vi "UDPSend.vi"(4 "error in (no error)":errorcluster, 6 "Data String":string="<data>", 8 "# Repetitions":i32=1, 9 "Remote Port":u16=1234, 10 "Local Port":u16=1233, 11 "Remote Host":string="localhost") -> (0 "error out":errorcluster)   [LabVIEW 2014]
doc: "This VI is designed to be used with the UDP Receiver VI. Run the UDP Receiver.vi first.\n\nThe UDP protocol differs from TCP in that there is no error-checking with the packets of information that are sent, and thus no guarantee whatsoever that an intended recipient will actually receive a given piece of data.\n\nUDP does offer the ability to \"broadcast\" data across a network--simply specify an IP Address of all ones (255.255.255.255) to attempt to broadcast information network-wide. Keep in mind that routers and other network hardware will generally refuse to forward the broadcast beyond certain points, so the extent of the broadcast will in practice be limited."
panel:
  in  "local Host":string="192.168.1.1"
  in  "broadcast":bool
  # "Instructions:\n1. Open the UDP Receiver.vi located in the same library.\n2. Make sure that the Remote Port in this VI and the Port in the UDP Receive.vi are the same.\n3. Press the button if you want to broadcast the data to all the network, instead of sending it to a specific address.\n4. Change the number of times you want to send the data to the receiver in the # of Repetitions control.\n5. Follow the instructions on it's front panel.\nNote: This VI is built to work with the UDP Receiver.vi."
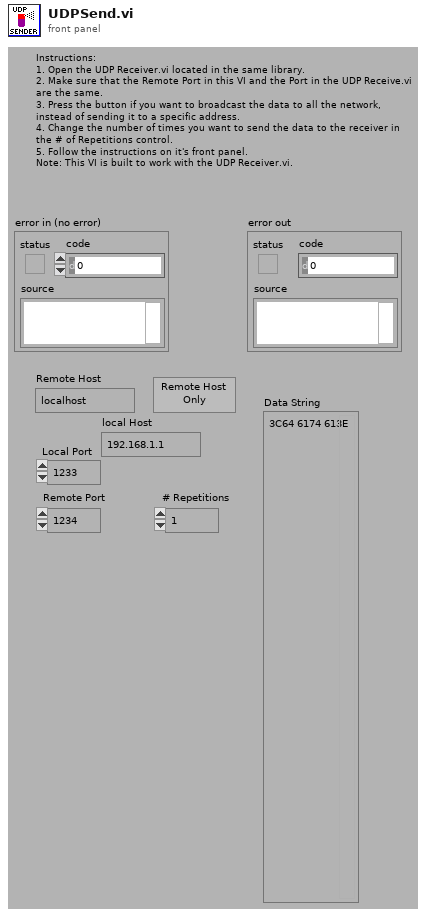
[diagram p1: front panel]
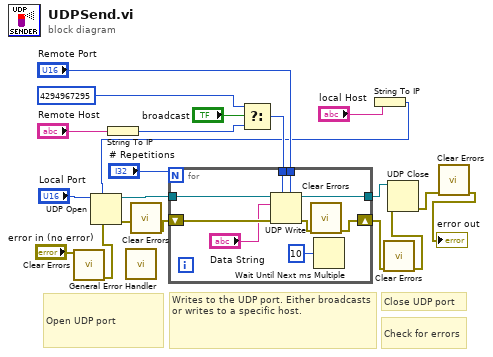
[diagram p0: block diagram]
diagram:
  # "Close UDP port"
  # "Check for errors"
  # "Writes to the UDP port. Either broadcasts or writes to a specific host."
  # "Open UDP port"
  n1 = call <vilib>:"Clear Errors.vi"("error in (no error)"="error in (no error)") -> ("error out"=w7:errorcluster)  [unwired: 1 in, 5 out]
  n2 = String To IP(1:"Remote Host") -> (0:w15:u32)
  n3 = call <vilib>:"General Error Handler.vi"() -> ()  [unwired: 3 in, 13 out]
  n4 = Select(t=u32 4294967295, s="broadcast", f=w15) -> (s? t:f=w14:u32)
  n5 = String To IP(1:"local Host") -> (0:w9:u32)
  n6 = UDP Open(7:w9, 8:w7, 11:"Local Port") -> (port=w20:refnum<k16>, 0:w4:errorcluster)  [unwired: 3 out]
  n7 = call <vilib>:"Clear Errors.vi"("error in (no error)"=w4) -> ("error out"=w3:errorcluster)  [unwired: 1 in, 5 out]
  n8 = for {
    N: "# Repetitions" -> [_]
    tunnel: w20 -> [w27]
    tunnel: w14 -> [w29]
    tunnel: "Remote Port" -> [w28]
    shift-right: [w21] -> w6
    shift-left: w3 -> [w26]
    tunnel: [w25] -> w18
    n9 = UDP Write(address=w29, port or service name=w28, connection ID=w27, data in="Data String", 8:w26) -> (error out=w22:errorcluster, 3:w25:refnum<k16>)  [unwired: 1 out]
    n10 = call <vilib>:"Clear Errors.vi"("error in (no error)"=w22) -> ("error out"=w21:errorcluster)  [unwired: 1 in, 5 out]
    n11 = Wait Until Next ms Multiple(millisecond multiple=u32 10) -> ()  [unwired: 1 out]
  }
  n12 = call <vilib>:"Clear Errors.vi"("error in (no error)"=w6) -> ("error out"=w5:errorcluster)  [unwired: 1 in, 5 out]
  n13 = UDP Close(connection ID=w18, 8:w5) -> (error out=w2:errorcluster)  [unwired: 1 out]
  n14 = call <vilib>:"Clear Errors.vi"("error in (no error)"=w2) -> ("error out"=→"error out":errorcluster)  [unwired: 1 in, 5 out]
